vi "GetAttributeViString.vi"(7 "AttributeValueBufferSize":i32=256, 8 "error in (no error)":errorcluster {"code" format="%.0x"}, 9 "AttributeID":u32(ring)=1150065 items=["CALIBRATION_DATE"=1150065, "CALIBRATION_MESSAGE"=1150015, "CALIBRATION_TIME"=1150066, "DIGITIZER_MEMORY_MEASUREMENT_DATA_AUTO_SAVE_FILE"=1150071, "DISPLAY_TEXT"=1150017, "DRIVER_SETUP"=1050007, "INSTRUMENT_FIRMWARE_REVISION"=1050510, "INSTRUMENT_MANUFACTURER"=1050511, "INSTRUMENT_MODEL"=1050512, "IO_RESOURCE_DESCRIPTOR"=1050304, "LOGICAL_NAME"=1050305, "ROUTE_MONITOR_CHANNEL"=1150010, "SCAN_LIST"=1150004, "SCAN_STARTTIME"=1150022, "SPECIFIC_DRIVER_DESCRIPTION"=1050514, "SPECIFIC_DRIVER_PREFIX"=1050302, "SPECIFIC_DRIVER_REVISION"=1050551, "SPECIFIC_DRIVER_VENDOR"=1050513, "SUPPORTED_INSTRUMENT_MODELS"=1050327, "SYSTEM_DATE"=1150020, "SYSTEM_SERIAL_NUMBER"=1150003, "SYSTEM_TIME"=1150021, "SYSTEM_TRACING_FILE_NAME"=1150042, "USB_MEMORY_DATA_FILE"=1150056, "USB_MEMORY_MEASUREMENTS_DATA_AUTO_SAVE_FILE"=1150058, "USB_MEMORY_SELECT_RECALL_AUTO_FILE"=1150053], 11 "instrument handle":refnum<k15>) -> (0 "error out":errorcluster {"code" format="%.0x"}, 2 "AttributeValue":string, 3 "instrument handle out":refnum<k15>)   [LabVIEW 2020, in "Keysight DAQ970.lvlib"]
doc: "Gets a String attribute from the instrument driver.\nThe following Attributes are supported:\n\nCALIBRATION_DATE\n\nCALIBRATION_MESSAGE\n\nCALIBRATION_TIME\n\nDIGITIZER_MEMORY_MEASUREMENT_DATA_AUTO_SAVE_FILE\n\nDISPLAY_TEXT\n\nDRIVER_SETUP\n\nINSTRUMENT_FIRMWARE_REVISION\n\nINSTRUMENT_MANUFACTURER\n\nINSTRUMENT_MODEL\n\nIO_RESOURCE_DESCRIPTOR\n\nLOGICAL_NAME\n\nROUTE_MONITOR_CHANNEL\n\nSCAN_LIST\n\nSCAN_STARTTIME\n\nSPECIFIC_DRIVER_DESCRIPTION\n\nSPECIFIC_DRIVER_PREFIX\n\nSPECIFIC_DRIVER_REVISION\n\nSPECIFIC_DRIVER_VENDOR\n\nSUPPORTED_INSTRUMENT_MODELS\n\nSYSTEM_DATE\n\nSYSTEM_SERIAL_NUMBER\n\nSYSTEM_TIME\n\nSYSTEM_TRACING_FILE_NAME\n\nUSB_MEMORY_DATA_FILE\n\nUSB_MEMORY_MEASUREMENTS_DATA_AUTO_SAVE_FILE\n\nUSB_MEMORY_SELECT_RECALL_AUTO_FILE"
uses:
  Keysight DAQ970.lvlib
  KtDAQ970.dll
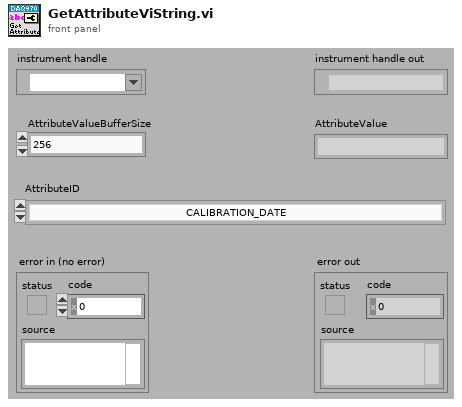
[diagram p1: front panel]
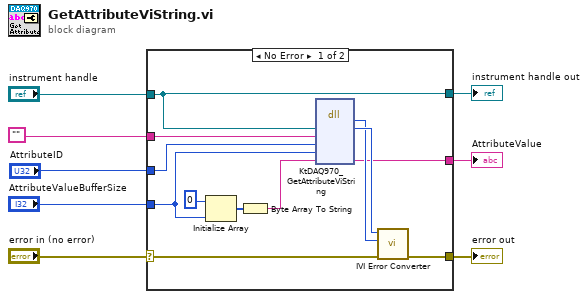
[diagram p0: block diagram]
diagram:
  n1 = case shown="No Error" "error in (no error)" {
    selector: "error in (no error)" -> [w18 w22]
    tunnel: [w17 w22] -> w8
    tunnel: "instrument handle" -> [w10 w21]
    tunnel: "" -> [w16 _]
    tunnel: "AttributeID" -> [w15 _]
    tunnel: "AttributeValueBufferSize" -> [w9 _]
    tunnel: [w11 _] -> w4
    tunnel: [w10 w21] -> w3
    frame No Error {
      n2 = Initialize Array(u8 0 ("element"), w9) -> (w13:u8[])
      n3 = Byte Array To String(unsigned byte array=w13) -> (string=w14:string)
      n4 = dll-call lib="KtDAQ970**.dll" fn="KtDAQ970_GetAttributeViString"("Vi"=w10, "RepCapIdentifier"=w16, "AttributeID"=w15, "AttributeValueBufferSize"=w9, "AttributeValue"=w14) -> ("return type"=w19:i32, "Vi"=w20:u32, "AttributeValue"=w11:string)  [unwired: 6 in, 2 out]
      n5 = call "IVI Error Converter.vi"("error in (no error)"=w18, "IVI error code (0)"=w19, "instrument handle"=w20) -> ("error out"=w17:errorcluster)  [unwired: 7 in, 1 out]
    }
    frame Error {
    }
  }
  "error out" <- w8
  "instrument handle out" <- w3
  "AttributeValue" <- w4
